vi "Teleop.vi"(10 "Match Info":T1={"Autonomous Elapsed Seconds"=0.0, "TeleOp Elapsed Seconds"=0.0, "Disabled Elapsed Seconds"=0.0, "Visited Autonomous"=FALSE, "Visited TeleOp"=FALSE, "Visited Disabled"=FALSE, "Autonomous Settings"={"Autonomous Style"=enum."Independent", "VI Refnum"=refnum}}, 11 "Call Context":T2) -> ()   [LabVIEW 2012]
doc: "This VI is called for each TeleOp packet received from the DS where the robot is not disabled. It is often used to read from the joysticks and update I/O or to update setpoints for timed control loops. It should complete and return within 20 milliseconds or it may miss DS packets."
uses:
  <vilib>/Rock Robotics/WPI/DriverStation/WPI_DriverStationDerivedRobotMode.ctl
  <vilib>/Rock Robotics/WPI/DriverStation/WPI_DriverStationMatch Info.ctl
  Robot Global Data.vi
  <vilib>/Rock Robotics/WPI/RobotDrive/WPI_RobotDriveMecanumDrive_Cartesian.vi
  <vilib>/Rock Robotics/WPI/RobotDrive/WPI_RobotDriveGetSetRefNum.vi
panel:
  in  "DeadZone":dbl=0.05
  in  "Apply PID":bool
  in  "D":dbl
  in  "I":dbl
  in  "P":dbl
  in  "Multiplier":dbl=1000.0
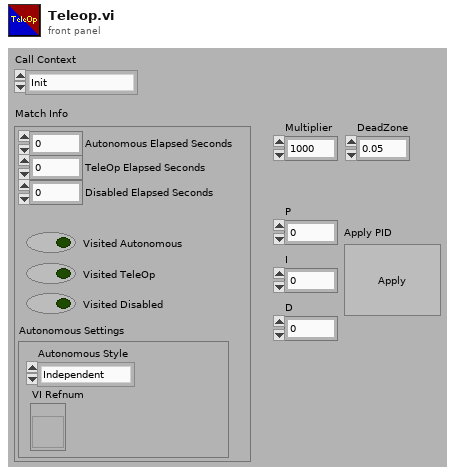
[diagram p1: front panel]
types:
  T1 = typedef "WPI_DriverStationMatch Info.ctl" = cluster{"Autonomous Elapsed Seconds":dbl, "TeleOp Elapsed Seconds":dbl, "Disabled Elapsed Seconds":dbl, "Visited Autonomous":bool, "Visited TeleOp":bool, "Visited Disabled":bool, "Autonomous Settings":cluster{"Autonomous Style":enum16{"Iterative", "Independent"}, "VI Refnum":refnum<vi>}}
  T2 = typedef "WPI_DriverStationDerivedRobotMode.ctl" = enum16{"Init", "Execute", "Stop"}
  T3 = cluster{"X":bool, "A":bool, "B":bool, "Y":bool, "LB":bool, "RB":bool, "LT":bool, "RT":bool, "Back":bool, "Start":bool, "LC":bool, "RC":bool}
  T4 = typedef "WPI_RobotDriveDevRef.ctl" = cluster{"DevStatus":errorcluster, "Motors[]":T5[], "Square Inputs":bool, "Max Output":dbl, "Isochronous":bool}
  T5 = typedef "WPI_MotorControlDeviceRef.ctl" = cluster{"DeviceStatus":errorcluster, "Type":enum16{"PWM", "CAN"}, "PWM":cluster{"Digital Module":T6, "PWM Channel":T7, "DeadBand":T8}, "CAN":cluster{"Device Number":u8, "Control Mode":T9, "Semaphore":T10, "Max Vout":dbl}, "Invert":bool, "TransformRef":T11, "InvTransformRef":T11}
  T6 = typedef "FPGA_TypedefDigitalModule.ctl" = enum16{"Digital Module 1", "Digital Module 2"}
  T7 = typedef "FPGA_DIOPWMChannel.ctl" = enum8{"PWM 1", "PWM 2", "PWM 3", "PWM 4", "PWM 5", "PWM 6", "PWM 7", "PWM 8", "PWM 9", "PWM 10", "Invalid"}
  T8 = typedef "WPI_PWMDeadband.ctl" = cluster{"Name":string, "maxPositivePwm":i32, "minPositivePwm":i32, "centerPwm":i32, "maxNegativePwm":i32, "minNegativePwm":i32, "angularRange":u16}
  T9 = typedef "WPI_CANJaguar_ControlMode.ctl" = enum8{"Percent VBus", "Current", "Speed", "Position", "Voltage"}
  T10 = typedef "Semaphore RefNum" = refnum<k1>
  T11 = typedef "WPI_PWMTransform_ConPane.ctl" = refnum<vi>
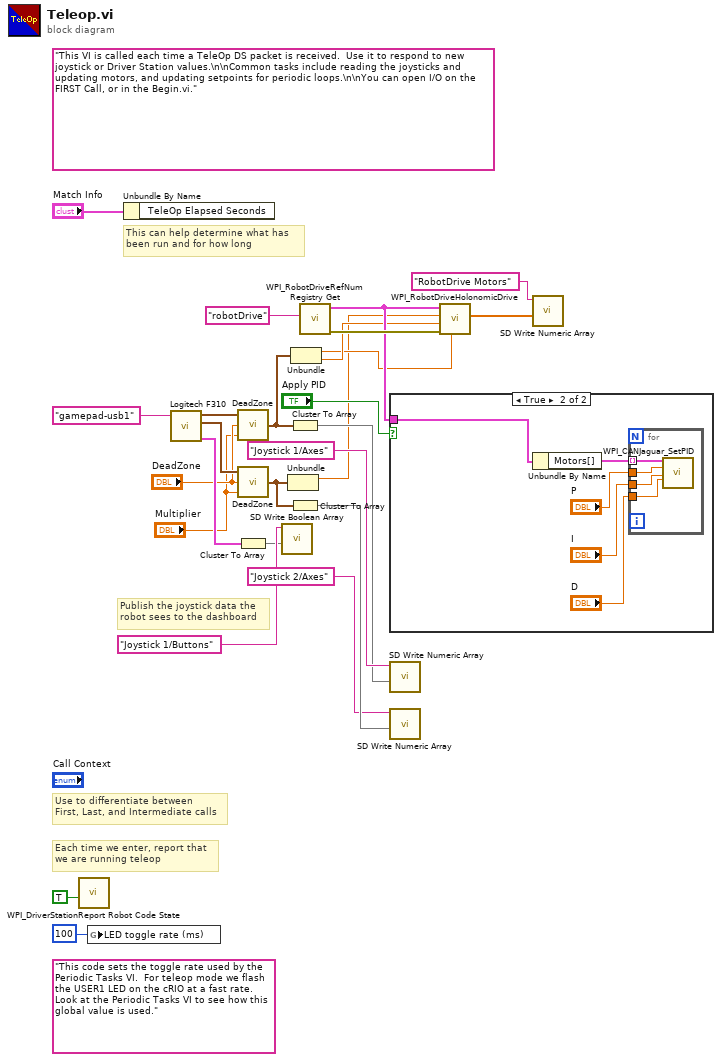
[diagram p0: block diagram]
diagram:
  (unwired) "This code sets the toggle rate used by the Periodic Tasks VI.  For teleop mode we flash the USER1 LED on the cRIO at a fast rate.  Look at the Periodic Tasks VI to see how this global value is used."
  (unwired) "This VI is called each time a TeleOp DS packet is received.  Use it to respond to new joystick or Driver Station values.\n\nCommon tasks include reading the joysticks and updating motors, and updating setpoints for periodic loops.\n\nYou can open I/O on the FIRST Call, or in the Begin.vi."
  # "Publish the joystick data the\nrobot sees to the dashboard"
  # "Each time we enter, report that\nwe are running teleop"
  # "Use to differentiate between\nFirst, Last, and Intermediate calls"
  # "This can help determine what has\nbeen run and for how long"
  n1 = call <vilib>:"WPI_DriverStationReport Robot Code State.vi"("TeleOp"=TRUE ("Autonomous")) -> ()  [unwired: 10 in, 1 out]
  n2 = global write "Robot Global Data.vi" "LED toggle rate (ms)"(u32 100 ("LED ms toggle rate")) -> ()
  n3 = Unbundle By Name("Match Info") -> ()  [unwired: 1 out]
  n4 = call "Logitech F310.vi"("refnum name"="gamepad-usb1") -> ("Buttons"=w13:T3, "Right Stick"=w10:cluster{"X":dbl, "Y":dbl}, "Left Stick"=w12:cluster{"X":dbl, "Y":dbl})  [unwired: 2 in, 3 out]
  n5 = call "DeadZone.vi"("Multiplier"="Multiplier", "DeadZone"="DeadZone", "Points(in)"=w12) -> ("Points(out)"=w11:cluster{"X":dbl, "Y":dbl})
  n6 = call "DeadZone.vi"("Multiplier"="Multiplier", "DeadZone"="DeadZone", "Points(in)"=w10) -> ("Points(out)"=w9:cluster{"X":dbl, "Y":dbl})
  n7 = Cluster To Array(cluster=w13) -> (array=w14:bool[])
  n8 = call <vilib>:"SD Write Boolean Array.vi"("Boolean Array"=w14, "Name"="Joystick 1/Buttons") -> ()  [unwired: 8 in, 2 out]
  n9 = Unbundle(w9) -> ("X"=w1:dbl)  [unwired: 1 out]
  n10 = Cluster To Array(cluster=w11) -> (array=w17:dbl[])
  n11 = Cluster To Array(cluster=w9) -> (array=w16:dbl[])
  n12 = Unbundle(w11) -> ("X"=w2:dbl, "Y"=w3:dbl)
  n13 = call <vilib>:"WPI_RobotDriveRefNum Registry Get.vi"("refnum name"="robotDrive") -> ("error out"=w18:errorcluster, "RobotDriveDevRef"=w5:T4)  [unwired: 1 in, 8 out]
  n14 = case shown="True" "Apply PID" {
    tunnel: w5 -> [_ w31]
    frame False {
    }
    frame True {
      n15 = Unbundle By Name(w31) -> ("Motors[]"=w30:T5[])
      n16 = for {
        tunnel: w30 -> [w35] mode=indexing
        tunnel: "P" -> [w34]
        tunnel: "I" -> [w33]
        tunnel: "D" -> [w32]
        n17 = call <vilib>:"WPI_CANJaguar_SetPID.vi"("CAN Jaguar Ref"=w35, "P"=w34, "I"=w33, "D"=w32) -> ()  [unwired: 10 in, 2 out]
      }
    }
  }
  n18 = call <vilib>:"SD Write Numeric Array.vi"("Numeric Array"=w17, "Name"="Joystick 1/Axes") -> ()  [unwired: 8 in, 2 out]
  n19 = call <vilib>:"SD Write Numeric Array.vi"("Numeric Array"=w16, "Name"="Joystick 2/Axes") -> ()  [unwired: 8 in, 2 out]
  n20 = call-poly <vilib>:"WPI_RobotDriveHolonomicDrive.vi"("Rotation"=w2, "error in (no error)"=w18, "Y"=w3, "X"=w1, "RobotDriveDevRef"=w5) -> ("Motor Values"=w20:dbl[])  [unwired: 4 in, 2 out]
  n21 = call <vilib>:"SD Write Numeric Array.vi"("Numeric Array"=w20, "Name"="RobotDrive Motors") -> ()  [unwired: 8 in, 2 out]
